vi "Drive Backwards.vi"() -> ()   [LabVIEW 2019]
uses:
  Robot Global Data.vi
panel:
  out "stop":bool
  in  "encoderDistance":dbl
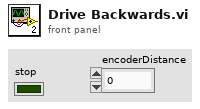
[diagram p1: front panel]
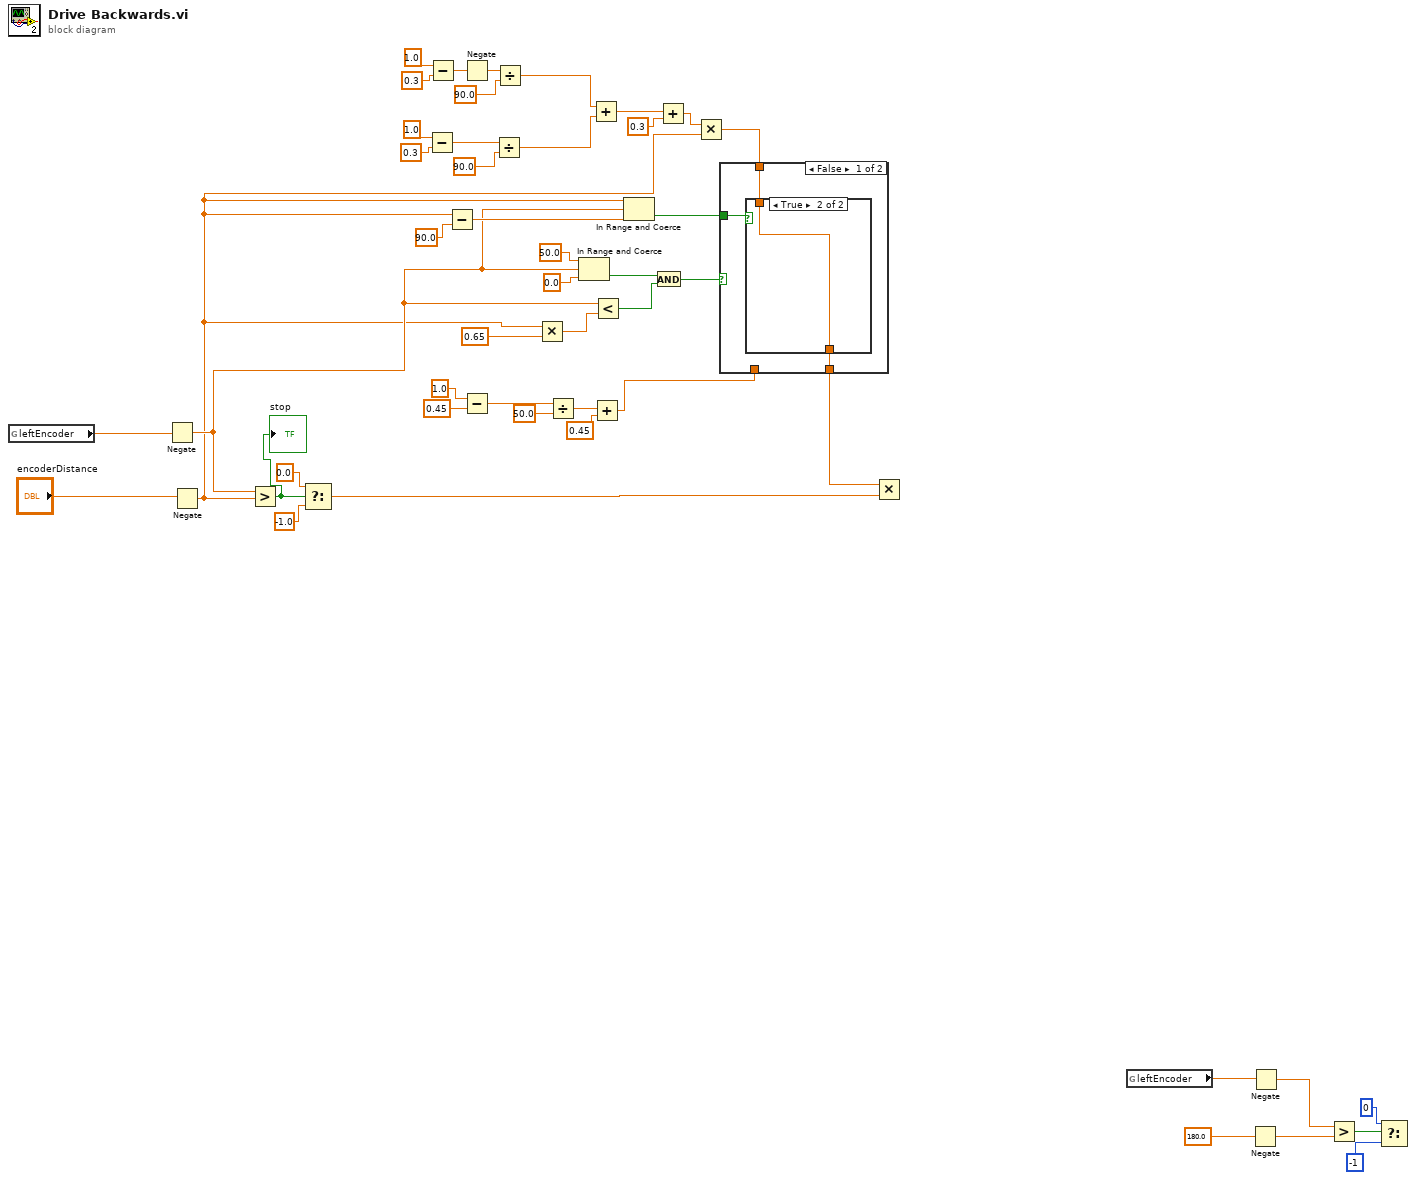
[diagram p0: block diagram]
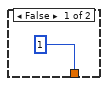
[diagram p2: hidden frame]
diagram:
  n1 = global read "Robot Global Data.vi" "leftEncoder"() -> (w41:dbl)
  n2 = Negate(x=w41) -> (-x=w26:dbl)
  n3 = Negate(x="encoderDistance") -> (-x=w5:dbl)
  n4 = Greater?(x=w26, y=w5) -> (0:w37:bool)
  "stop" <- w37
  n5 = Select(t=0.0, s=w37, f=-1.0) -> (s? t:f=w24:dbl)
  n6 = Subtract(x=1.0, y=0.3) -> (x-y=w11:dbl)
  n7 = Subtract(x=1.0, y=0.3) -> (x-y=w17:dbl)
  n8 = Subtract(x=w5, y=90.0) -> (x-y=w28:dbl)
  n9 = Negate(x=w17) -> (-x=w16:dbl)
  n10 = Subtract(x=1.0, y=0.45) -> (x-y=w22:dbl)
  n11 = Divide(x=w11, y=90.0) -> (x/y=w10:dbl)
  n12 = Divide(x=w16, y=90.0) -> (x/y=w9:dbl)
  n13 = Multiply(x=w5, y=0.65) -> (x*y=w35:dbl)
  n14 = Divide(x=w22, y=50.0) -> (x/y=w21:dbl)
  n15 = In Range and Coerce(upper limit=50.0, x=w26, lower limit=0.0) -> (In Range?=w33:bool)  [unwired: 1 out]
  n16 = Add(x=w9, y=w10) -> (x+y=w8:dbl)
  n17 = Add(x=w21, y=0.45) -> (x+y=w20:dbl)
  n18 = Less?(x=w26, y=w35) -> (x < y?=w34:bool)
  n19 = In Range and Coerce(upper limit=w5, x=w26, lower limit=w28) -> (In Range?=w27:bool)  [unwired: 1 out]
  n20 = And(x=w33, y=w34) -> (x .and. y?=w30:bool)
  n21 = Add(x=w8, y=0.3) -> (x+y=w6:dbl)
  n22 = Multiply(x=w6, y=w5) -> (x*y=w4:dbl)
  n23 = case shown="False" w30 {
    tunnel: w27 -> [w51 _]
    tunnel: [w50 w54] -> w25
    tunnel: w20 -> [_ w54]
    tunnel: w4 -> [w49 _]
    frame False {
      n24 = case shown="True" w51 {
        tunnel: [1 w53] -> w50
        tunnel: w49 -> [_ w53]
        frame False {
        }
        frame True {
        }
      }
    }
    frame True {
    }
  }
  n25 = Multiply(x=w25, y=w24) -> ()  [unwired: 1 out]
  n26 = global read "Robot Global Data.vi" "leftEncoder"() -> (w42:dbl)
  n27 = Negate(x=180.0) -> (-x=w45:dbl)
  n28 = Negate(x=w42) -> (-x=w44:dbl)
  n29 = Greater?(x=w44, y=w45) -> (0:w46:bool)
  n30 = Select(t=0, s=w46, f=-1) -> ()  [unwired: 1 out]
